vi "SyncLoopHandler.vi"(8 "error in (no error)":errorcluster, 10 "LoopProperties":refnum<class "SyncPluginBase.lvclass">, 11 "SyncPluginBase in":refnum<class "SyncPluginBase.lvclass">) -> (0 "error out":errorcluster, 3 "SyncPluginBase out":refnum<class "SyncPluginBase.lvclass">)   [LabVIEW 2014, in "SyncPlugins.lvlib" / "SyncPluginBase.lvclass"]
uses:
  SyncPluginBase.lvclass
  SyncPluginBase.lvclass/SyncPluginBase.ctl
  Accessors/Read Initiated.vi
  Accessors/Read Locked.vi
  Accessors/Read LostLock.vi
  Accessors/Read Monitor Loop.vi
  Accessors/Read PPSTime.vi
  Accessors/Read Run.vi
  Accessors/Write Initiated.vi
  Accessors/Write Locked.vi
  Accessors/Write LostLock.vi
  Accessors/Write Monitor Loop.vi
  Accessors/Write PPSTime.vi
  Accessors/Write Run.vi
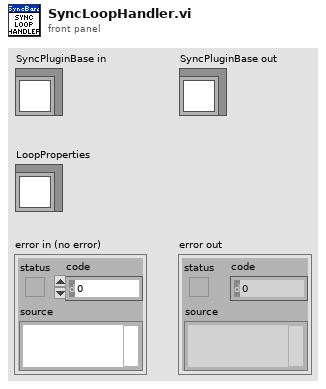
[diagram p1: front panel]
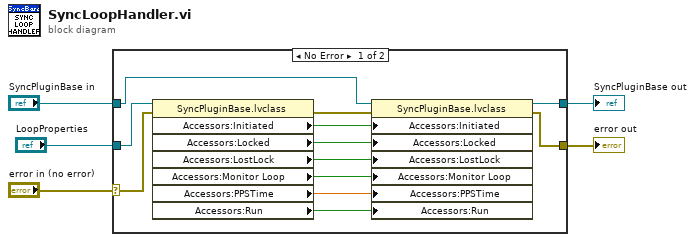
[diagram p0: block diagram]
diagram:
  n1 = case shown="No Error" "error in (no error)" {
    selector: "error in (no error)" -> [w10 w19]
    tunnel: [w8 w19] -> w4
    tunnel: [w17 w18] -> w2
    tunnel: "SyncPluginBase in" -> [w7 w18]
    tunnel: "LoopProperties" -> [w6 _]
    frame No Error {
      n2 = property class="SyncPluginBase.lvclass"(reference=w6, error in=w10) -> (error out=w9:errorcluster, "Accessors:Initiated"=w16:bool, "Accessors:Locked"=w15:bool, "Accessors:LostLock"=w14:bool, "Accessors:Monitor Loop"=w13:bool, "Accessors:PPSTime"=w12:dbl, "Accessors:Run"=w11:bool)  [unwired: 1 out]
      n3 = property class="SyncPluginBase.lvclass"(reference=w7, error in=w9, "Accessors:Initiated"=w16, "Accessors:Locked"=w15, "Accessors:LostLock"=w14, "Accessors:Monitor Loop"=w13, "Accessors:PPSTime"=w12, "Accessors:Run"=w11) -> (reference out=w17:refnum<class "SyncPluginBase.lvclass">, error out=w8:errorcluster)
    }
    frame Error {
    }
  }
  "error out" <- w4
  "SyncPluginBase out" <- w2
